vi "Remove SR Popup.vi"(8 "error in":errorcluster, 9 "Monitor":u16) -> (0 "error out":errorcluster, 3 "SR array out":i32[](array[numeric]))   [LabVIEW 2018]
uses:
  <vilib>/Utility/miscctls.llb/LVPointTypeDef.ctl
panel:
  in  "Close":bool
  in  "Remove SR":bool
  in  "SR to Remove":string
  # "Enter SR number(s) seperated by commas,\n press \"Remove SRs\" to take it from the list"
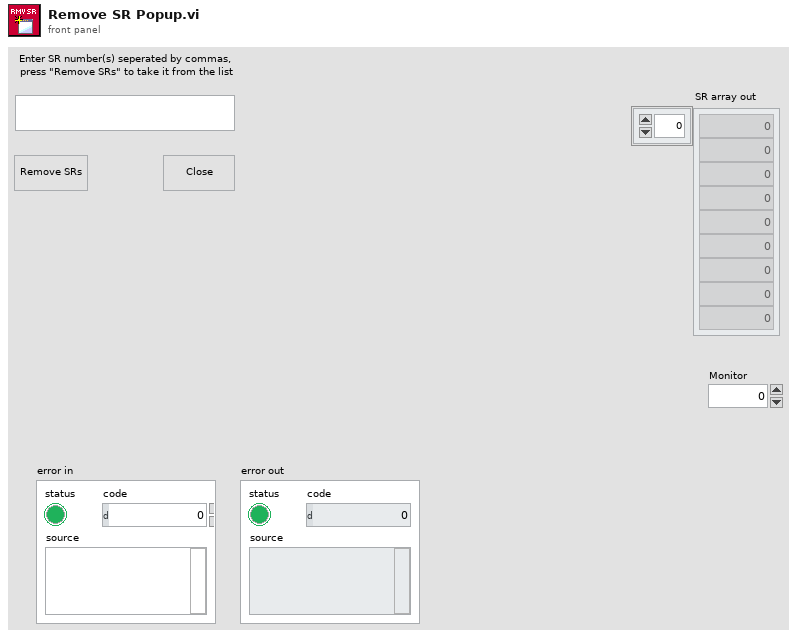
[diagram p1: front panel]
types:
  T1 = typedef "LVPointTypeDef.ctl" = cluster{"Horizontal":i16, "Vertical":i16}
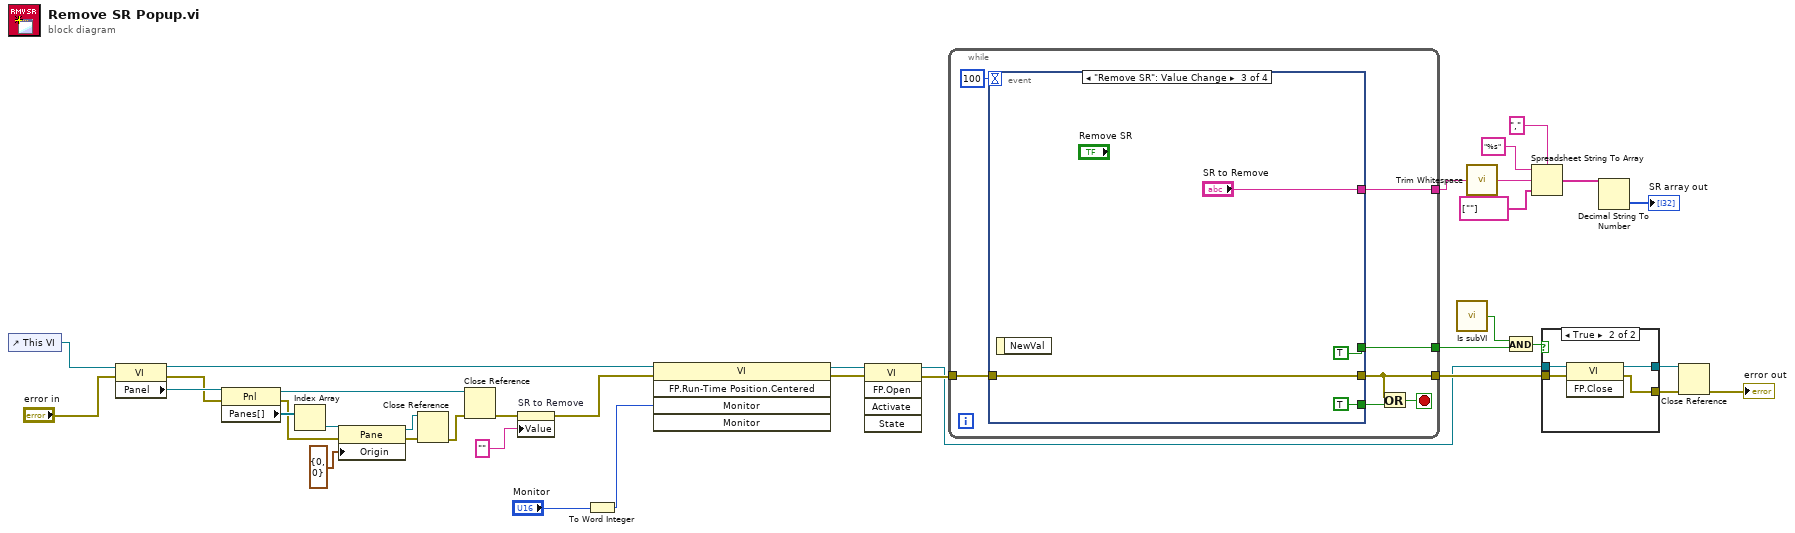
[diagram p0: block diagram]
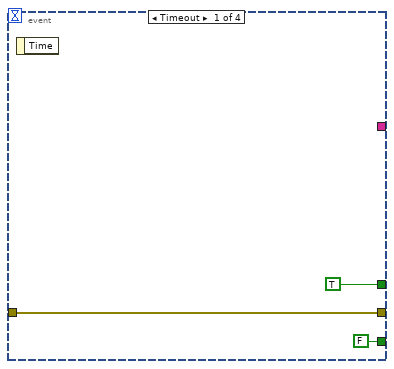
[diagram p3: hidden frame]
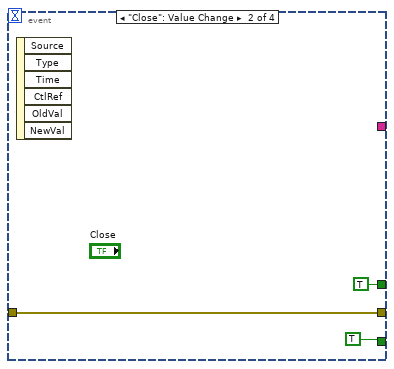
[diagram p4: hidden frame]
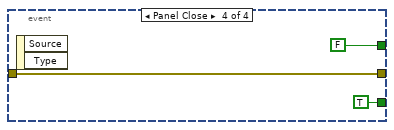
[diagram p5: hidden frame]
diagram:
  n1 = control-ref of="This VI"() -> (w12:refnum<vi>)
  n2 = property class="VI"(reference=w12, error in="error in") -> (reference out=w3:refnum<vi>, error out=w13:errorcluster, "Panel"=w14:refnum<vi>)
  n3 = property class="Pnl"(reference=w14, error in=w13) -> (reference out=w15:refnum<vi>, error out=w20:errorcluster, "Panes[]"=w22:refnum<vi>[])
  n4 = Index Array(array=w22) -> (element=w21:refnum<vi>)  [unwired: 1 in]
  n5 = property class="Pane"(reference=w21, error in=w20, "Origin"=T1 {"Horizontal"=0, "Vertical"=0}) -> (reference out=w18:refnum<vi>, error out=w17:errorcluster)
  n6 = Close Reference(reference=w18, error in (no error)=w17) -> (error out=w16:errorcluster)
  n7 = Close Reference(reference=w15, error in (no error)=w16) -> (error out=w9:errorcluster)
  n8 = property on="SR to Remove" class="Str"(error in=w9, "Value"="" ("SR to Remove")) -> (error out=w5:errorcluster)  [unwired: 1 in, 1 out]
  n9 = To Word Integer(number="Monitor") -> (16bit integer=w1:i16)
  n10 = invoke class="VI" method="FP.Run-Time Position.Centered"(reference=w3, error in=w5, "Monitor"=w1) -> (reference out=w7:refnum<vi>, error out=w6:errorcluster)  [unwired: 2 in, 3 out]
  n11 = invoke class="VI" method="FP.Open"(reference=w7, error in=w6) -> (reference out=w10:refnum<vi>, error out=w11:errorcluster)  [unwired: 3 in, 3 out]
  n12 = while {
    tunnel: w11 -> [w41]
    tunnel: [w39] -> w36
    tunnel: [w42] -> w24
    tunnel: [w37] -> w31
    stop <- w40 stop-if-true
    n13 = event shown="[2] \"Remove SR\": Value Change" {
      selector: _ -> [_ _ _ _]
      dyn-events: _ -> [_ _ _ _]
      timeout: 100 -> [_ _ _ _]
      tunnel: w41 -> [w45 w47 w53 w56]
      tunnel: [w45 w47 w53 w56] -> w39
      tunnel: [TRUE TRUE TRUE FALSE] -> w42
      tunnel: [FALSE TRUE TRUE TRUE] -> w38
      tunnel: [_ _ "SR to Remove" _] -> w37
      event Timeout {
        n14 = event-data() -> ()  [unwired: 1 in, 1 out]
      }
      event "Close": Value Change {
        n15 = event-data() -> ()  [unwired: 1 in, 6 out]
      }
      event "Remove SR": Value Change {
        n16 = event-data() -> ()  [unwired: 1 in, 1 out]
      }
      event Panel Close {
        n17 = event-data() -> ()  [unwired: 1 in, 2 out]
      }
    }
    n18 = Or(x=w39, y=w38) -> (x .or. y?=w40:bool)
  }
  n19 = call "Is subVI.vi"() -> ("Is subVI?"=w23:bool)  [unwired: 1 in]
  n20 = call <vilib>:"Trim Whitespace.vi"("string"=w31) -> ("trimmed string"=w30:string)  [unwired: 1 in]
  n21 = And(x=w23, y=w24) -> (x .and. y?=w25:bool)
  n22 = Spreadsheet String To Array(delimiter (Tab)=",", format string="%s", spreadsheet string=w30, array type (2D Dbl)=string[] [""]) -> (array=w27:string[])
  n23 = case shown="True" w25 {
    tunnel: w10 -> [w58 w62]
    tunnel: w36 -> [w57 w61]
    tunnel: [w58 w60] -> w35
    tunnel: [w57 w59] -> w34
    frame False {
    }
    frame True {
      n24 = invoke class="VI" method="FP.Close"(reference=w62, error in=w61) -> (reference out=w60:refnum<vi>, error out=w59:errorcluster)  [unwired: 1 in, 1 out]
    }
  }
  n25 = Decimal String To Number(string=w27) -> (number=→"SR array out":i32[])  [unwired: 2 in, 1 out]
  n26 = Close Reference(reference=w35, error in (no error)=w34) -> (error out=→"error out":errorcluster)
